vi "Extract IRF (Direct).vi"(4 "balance parameter (-1: auto)":dbl=-1.0, 5 "Period":dbl, 6 "Tail Smoothing (T)":bool=TRUE, 7 "Smoothing Order":i32=1, 8 "Error In":errorcluster, 9 "Time Constant":dbl, 10 "Intensity Array":dbl[](array[numeric]), 11 "t Array":dbl[](array[numeric])) -> (0 "Error Out":errorcluster, 1 "Message":string, 2 "IRF Array":dbl[](array[numeric]), 3 "t Array (dup)":dbl[](array[numeric]))   [LabVIEW 2021, in "Fits.lvlib"]
doc: "Extract IRF from provided decay and time constant"
uses:
  Fits.lvlib
  Graphs/XY Graph/XY Graph Add-Ons.lvlib
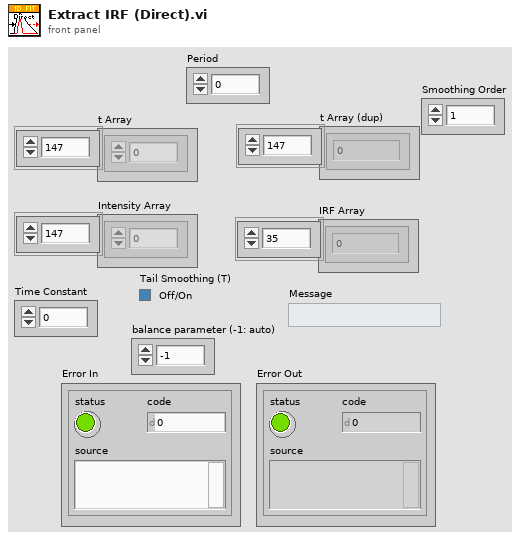
[diagram p1: front panel]
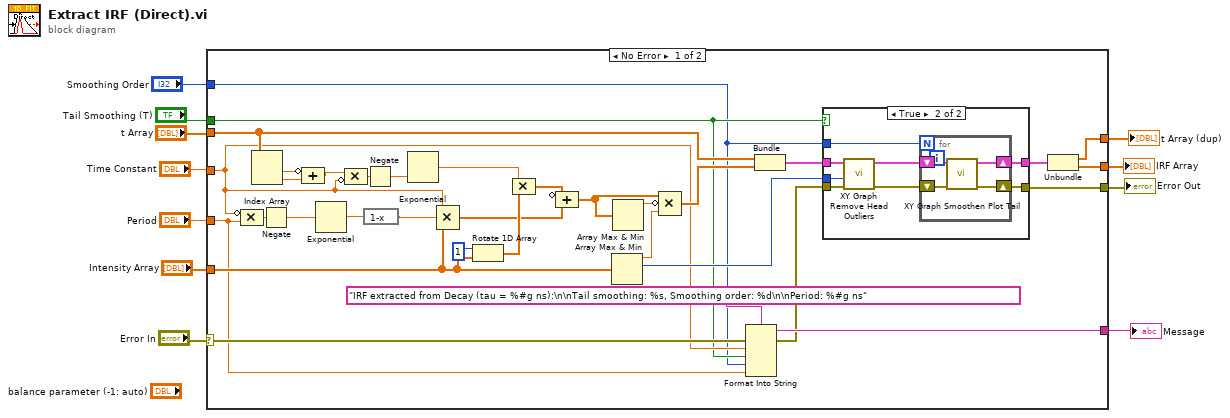
[diagram p0: block diagram]
diagram:
  n1 = case shown="No Error" "Error In" {
    selector: "Error In" -> [w43 w60]
    tunnel: "Intensity Array" -> [w27 _]
    tunnel: "Time Constant" -> [w21 _]
    tunnel: "t Array" -> [w26 _]
    tunnel: [w42 w60] -> w8
    tunnel: [w44 _] -> w6
    tunnel: "Tail Smoothing (T)" -> [w14 _]
    tunnel: [w40 _] -> w4
    tunnel: [w39 _] -> w3
    tunnel: "Smoothing Order" -> [w13 _]
    tunnel: "Period" -> [w12 _]
    frame No Error {
      n2 = Compound Arithmetic op=MULTIPLY(invert w21, w12) -> (w31:dbl)
      n3 = Index Array(array=w26) -> (element #1=w25:dbl, element #2=w24:dbl)  [unwired: 2 in]
      n4 = Negate(x=w31) -> (-x=w28:dbl)
      n5 = Compound Arithmetic op=ADD(invert w25, w24) -> (w22:dbl)
      n6 = Exponential(1:w28) -> (0:w30:dbl)
      n7 = Compound Arithmetic op=MULTIPLY(w22, invert w21) -> (w23:dbl)
      n8 = expression code="1-x"(w30) -> (w29:dbl)
      n9 = Negate(x=w23) -> (-x=w20:dbl)
      n10 = Exponential(1:w20) -> (0:w45:dbl)
      n11 = Compound Arithmetic op=MULTIPLY(w21, w29, w27) -> (w17:dbl[])
      n12 = Rotate 1D Array(1:w27, 2:1 ("n")) -> (0:w19:dbl[])
      n13 = Compound Arithmetic op=MULTIPLY(w45, w19) -> (w18:dbl[])
      n14 = Compound Arithmetic op=ADD(invert w18, w17) -> (w15:dbl[])
      n15 = Array Max & Min(array=w27) -> (max value=w38:dbl, max index (indices)=w34:i32)  [unwired: 2 out]
      n16 = Array Max & Min(array=w15) -> (max value=w16:dbl)  [unwired: 3 out]
      n17 = Compound Arithmetic op=MULTIPLY(w15, invert w16, w38) -> (w36:dbl[])
      n18 = Format Into String(format string="IRF extracted from Decay (tau = %#g ns):\n\nTail smoothing: %s, Smoothing order: %d\n\nPeriod: %#g ns" ("Message"), error in=w43, w21, w14, w13, w12) -> (resulting string=w44:string, error out=w33:errorcluster)  [unwired: 1 in]
      n19 = Bundle("t Array"=w26, w36) -> (w35:cluster{"t Array":dbl[], dbl[]})  [unwired: 1 in]
      n20 = case shown="True" w14 {
        tunnel: w34 -> [_ w51]
        tunnel: w35 -> [w46 w48]
        tunnel: [w46 w55] -> w41
        tunnel: w33 -> [w47 w49]
        tunnel: [w47 w54] -> w42
        tunnel: w13 -> [_ w53]
        frame False {
        }
        frame True {
          n21 = call "XY Graph Remove Head Outliers.vi"("Error In"=w49, "Peak Index (-1: unknown)"=w51, "Plot in"=w48) -> ("Error Out"=w50:errorcluster, "Plot out"=w52:cluster{"t Array":dbl[], "Array":dbl[]})  [unwired: 6 in, 1 out]
          n22 = for {
            N: w53 -> [_]
            shift-right: [w57] -> w55
            shift-left: w52 -> [w59]
            shift-right: [w56] -> w54
            shift-left: w50 -> [w58]
            n23 = call "XY Graph Smoothen Plot Tail.vi"("error in (no error)"=w58, "Plot in"=w59) -> ("error out"=w56:errorcluster, "Plot out"=w57:cluster{"t Array":dbl[], "Y Array":dbl[]})  [unwired: 8 in]
          }
        }
      }
      n24 = Unbundle(w41) -> ("t Array"=w40:dbl[], "Array"=w39:dbl[])
    }
    frame Error {
    }
  }
  "IRF Array" <- w3
  "Error Out" <- w8
  "t Array (dup)" <- w4
  "Message" <- w6
